vi "Autonomous_Execution.vi"(0 "Queue Key":refnum<queue>, 5 "Autonomous_Queue":refnum<queue>, 11 "error in":errorcluster) -> (6 "Done":bool)   [LabVIEW 2020]
uses:
  Globals/Drive_Globals.vi
  Queue_Key_Data.ctl
  Subsystems/Drive/Drive_Control_States.ctl
  Subsystems/Drive/Drive_Orientation_States.ctl
  Subsystems/Drive/Drive_Cluster.ctl
  Robot_Subsystems.ctl
panel:
  in  "ignore previous (F)":bool
  in  "timeout in ms (-1)":i32=15
  out "notifiers out":refnum<notifier>[](array[refnum])
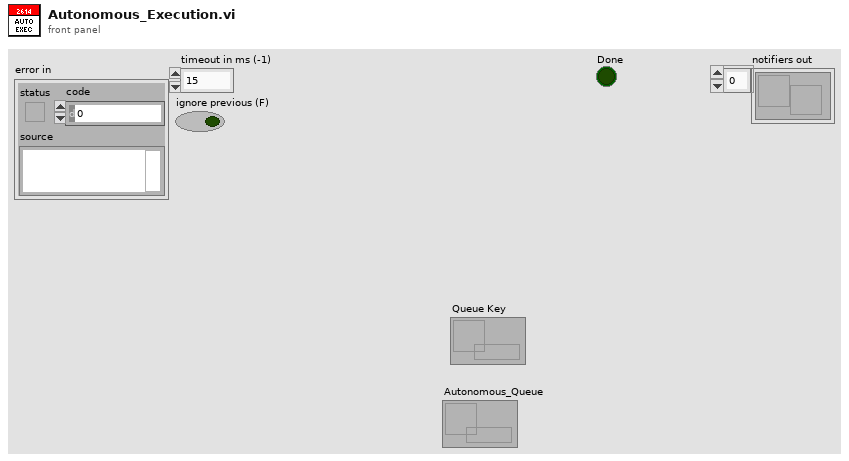
[diagram p1: front panel]
types:
  T1 = typedef "Queue_Key_Data.ctl" = cluster{"Operation Notifier":refnum<notifier>, "Subsystem":string, "Concurrent":bool}
  T2 = typedef "Robot_Subsystems.ctl" = cluster{"Drive_Cluster":T3}
  T3 = typedef "Drive_Cluster.ctl" = cluster{"Control_State":T4, "Vertical_Throttle":dbl, "Lateral_Throttle":dbl, "Rotational_Throttle":dbl, "Strafe_In_Deadband":bool, "Rotation_In_Deadband":bool, "Orientation_State":T5, "Parameters":dbl[], "Step":i32, "Auto_Notifier":refnum<notifier>, "PathName":string}
  T4 = typedef "Drive_Control_States.ctl" = enum16{"No-Op", "Manual_Control", "Command_DriveDistanceAtAngle", "Command_DrivePath", "Command_SetRobotPose"}
  T5 = typedef "Drive_Orientation_States.ctl" = enum16{"Robot-Oriented", "Field-Oriented"}
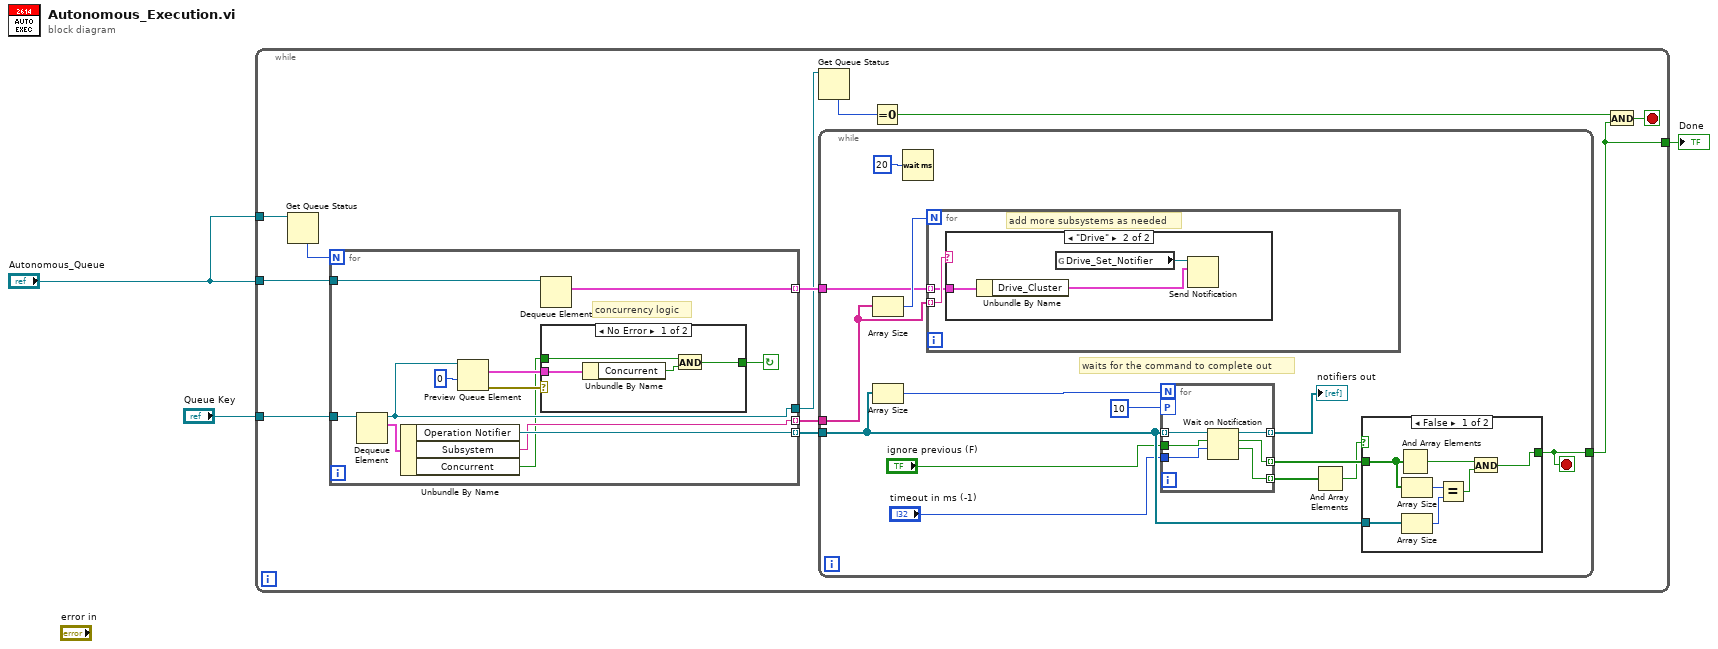
[diagram p0: block diagram]
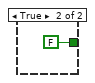
[diagram p2: hidden frame]
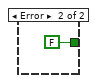
[diagram p4: hidden frame]
diagram:
  n1 = while {
    tunnel: "Queue Key" -> [w14]
    tunnel: "Autonomous_Queue" -> [w15]
    tunnel: "Autonomous_Queue" -> [w6]
    tunnel: [w4] -> w2
    stop <- w7 stop-if-true
    n2 = Get Queue Status(queue=w6) -> (# elements in queue=w9:i32)  [unwired: 2 in, 7 out]
    n3 = for {
      N: w9 -> [_]
      tunnel: w15 -> [w54]
      tunnel: w14 -> [w60]
      tunnel: [w51] -> w10 mode=indexing
      tunnel: [w55] -> w5
      tunnel: [w50] -> w12 mode=indexing
      tunnel: [w53] -> w11 mode=indexing
      stop <- w56 continue-if-true
      # "concurrency logic"
      n4 = Dequeue Element(queue=w60) -> (queue out=w55:refnum<queue>, element=w52:T1)  [unwired: 2 in, 2 out]
      n5 = Unbundle By Name(w52) -> ("Operation Notifier"=w51:refnum<notifier>, "Subsystem"=w50:string, "Concurrent"=w49:bool)
      n6 = Preview Queue Element(queue=w55, timeout in ms (-1)=0) -> (element=w59:T1, error out=w57:errorcluster)  [unwired: 1 in, 2 out]
      n7 = Dequeue Element(queue=w54) -> (element=w53:T2)  [unwired: 2 in, 3 out]
      n8 = case shown="No Error" w57 {
        tunnel: w59 -> [w62 _]
        tunnel: [w64 FALSE] -> w56
        tunnel: w49 -> [w63 _]
        frame No Error {
          n9 = Unbundle By Name(w62) -> ("Concurrent"=w61:bool)
          n10 = And(x=w63, y=w61) -> (x .and. y?=w64:bool)
        }
        frame Error {
        }
      }
    }
    n11 = Get Queue Status(queue=w5) -> (# elements in queue=w13:i32)  [unwired: 2 in, 7 out]
    n12 = while {
      tunnel: w12 -> [w24]
      tunnel: w11 -> [w23]
      tunnel: w10 -> [w25]
      tunnel: [w26] -> w4
      stop <- w26 stop-if-true
      # "waits for the command to complete out"
      n13 = Array Size(array=w24) -> (size(s)=w27:i32)
      n14 = Array Size(array=w25) -> (size(s)=w19:i32)
      n15 = Wait (ms)(milliseconds to wait=u32 20) -> ()  [unwired: 1 out]
      n16 = for {
        N: w27 -> [_]
        tunnel: w24 -> [w45] mode=indexing
        tunnel: w23 -> [w44] mode=indexing
        # "add more subsystems as needed"
        n17 = case shown="\"Drive\"" w45 {
          tunnel: w44 -> [_ w48]
          frame "No_Op", Default {
          }
          frame "Drive" {
            n18 = Unbundle By Name(w48) -> ("Drive_Cluster"=w47:T3)
            n19 = global read "Drive_Globals.vi" "Drive_Set_Notifier"() -> (w46:refnum<notifier>)
            n20 = Send Notification(notification=w47, notifier=w46) -> ()  [unwired: 1 in, 2 out]
          }
        }
      }
      n21 = for {
        N: w19 -> [_]
        tunnel: w25 -> [w35] mode=indexing
        workers-P: 10 -> [_]
        tunnel: "timeout in ms (-1)" -> [w34]
        tunnel: "ignore previous (F)" -> [w33]
        tunnel: [w32] -> w22 mode=indexing
        tunnel: [w31] -> w29 mode=indexing
        tunnel: [w30] -> w17 mode=indexing
        n22 = Wait on Notification(notifier=w35, ignore previous (F)=w33, timeout in ms (-1)=w34) -> (notifier out=w32:refnum<notifier>, notification=w31:bool, timed out?=w30:bool)  [unwired: 1 in, 1 out]
      }
      "notifiers out" <- w22
      n23 = And Array Elements(Boolean array=w17) -> (logical AND=w28:bool)
      n24 = case shown="False" w28 {
        tunnel: [w41 FALSE] -> w26
        tunnel: w29 -> [w40 _]
        tunnel: w25 -> [w39 _]
        frame False {
          n25 = And Array Elements(Boolean array=w40) -> (logical AND=w42:bool)
          n26 = Array Size(array=w40) -> (size(s)=w38:i32)
          n27 = Array Size(array=w39) -> (size(s)=w37:i32)
          n28 = Equal?(x=w38, y=w37) -> (x = y?=w36:bool)
          n29 = And(x=w42, y=w36) -> (x .and. y?=w41:bool)
        }
        frame True {
        }
      }
    }
    n30 = Equal To 0?(x=w13) -> (x = 0?=w8:bool)
    n31 = And(x=w8, y=w4) -> (x .and. y?=w7:bool)
  }
  "Done" <- w2
